vi "Visit Me.vi"(8 "error in (no error)":errorcluster, 10 "Visitor In":refnum<class "LVTypeVisitor.lvclass">, 11 "LVClusterType in":refnum<class "LVClusterType.lvclass">) -> (0 "error out":errorcluster, 2 "Visitor Out":refnum<class "LVTypeVisitor.lvclass">, 3 "LVClusterType out":refnum<class "LVClusterType.lvclass">)   [LabVIEW 2020, in "LVDataTypes.lvlib" / "LVClusterType.lvclass"]
uses:
  <vilib>/AppBuilder/Engine/WebServiceDescription/LVDataTypes/LVClusterType/LVClusterType.lvclass
  <vilib>/AppBuilder/Engine/WebServiceDescription/LVDataTypes/LVTypeVisitor/LVTypeVisitor.lvclass
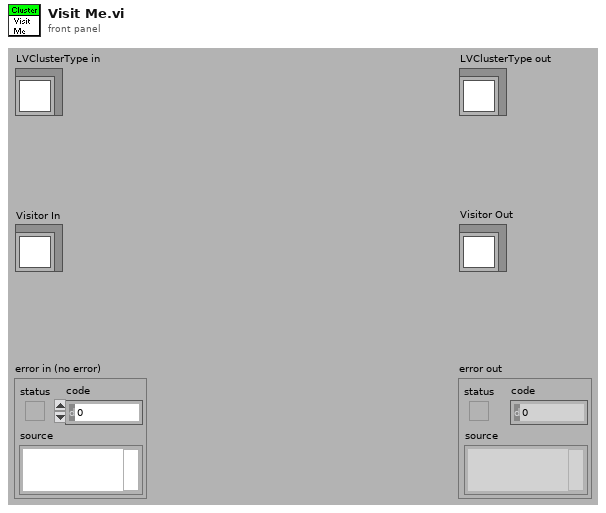
[diagram p1: front panel]
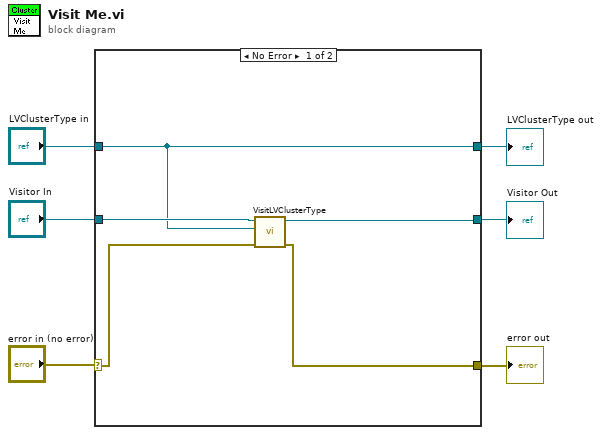
[diagram p0: block diagram]
diagram:
  n1 = case shown="No Error" "error in (no error)" {
    selector: "error in (no error)" -> [w10 w14]
    tunnel: [w9 w14] -> w5
    tunnel: [w7 w13] -> w3
    tunnel: "Visitor In" -> [w11 w13]
    tunnel: [w8 w12] -> w1
    tunnel: "LVClusterType in" -> [w8 w12]
    frame No Error {
      n2 = call-dynamic "VisitLVClusterType.vi"("error in (no error)"=w10, "LVClusterType"=w8, "LVTypeVisitor in"=w11) -> ("error out"=w9:errorcluster, "LVTypeVisitor out"=w7:refnum<class "LVTypeVisitor.lvclass">)  [unwired: 7 out]
    }
    frame Error {
    }
  }
  "error out" <- w5
  "LVClusterType out" <- w1
  "Visitor Out" <- w3
